vi "Write Controls.vi"(8 "error in (no error)":errorcluster, 10 "Controls":T1(array[cluster])=[{"Ring 2"=refnum, "Sub Panel 2"=refnum}, {"Ring 2"=refnum, "Sub Panel 2"=refnum}], 11 "Test.Maui 2.0.Panels in":refnum<class "Test.Maui 2.0.Panels.lvclass">) -> (0 "error out":errorcluster, 3 "Test.Maui 2.0.Panels out":refnum<class "Test.Maui 2.0.Panels.lvclass">)   [LabVIEW 2020, in "Test.Maui 2.0.Panels.lvclass"]
uses:
  Test.Maui 2.0.Panels.lvclass
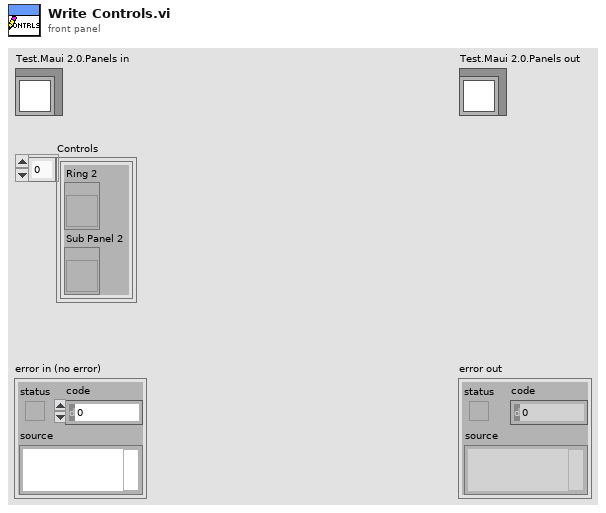
[diagram p1: front panel]
types:
  T1 = cluster{"Ring 2":refnum<vi>, "Sub Panel 2":refnum<vi>}[]
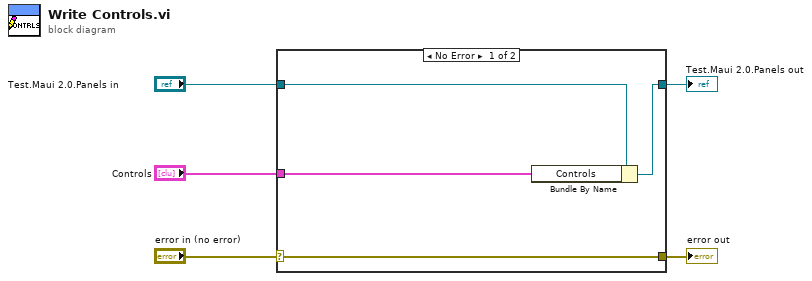
[diagram p0: block diagram]
diagram:
  n1 = case shown="No Error" "error in (no error)" {
    selector: "error in (no error)" -> [w9 w10]
    tunnel: [w9 w10] -> w4
    tunnel: [w7 w11] -> w2
    tunnel: "Test.Maui 2.0.Panels in" -> [w8 w11]
    tunnel: "Controls" -> [w6 _]
    frame No Error {
      n2 = Bundle By Name(cluster=w8, "Controls"=w6) -> (w7:refnum<class "Test.Maui 2.0.Panels.lvclass">)
    }
    frame Error {
    }
  }
  "error out" <- w4
  "Test.Maui 2.0.Panels out" <- w2
